vi "ImportConfigFile.vi"(4 "error in (no error)":errorcluster, 5 "bVerify":bool=TRUE, 6 "pszFilePath":string, 7 "nInputHandle":u64) -> (0 "error out":errorcluster, 1 "GX_STATUS":i32, 3 "nOutputHandle":u64)   [LabVIEW 2016, in "GxLVLib.lvlib"]
uses:
  GxLVLib.lvlib
  GxIAPI.dll
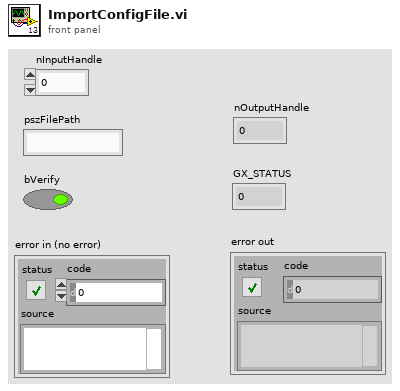
[diagram p1: front panel]
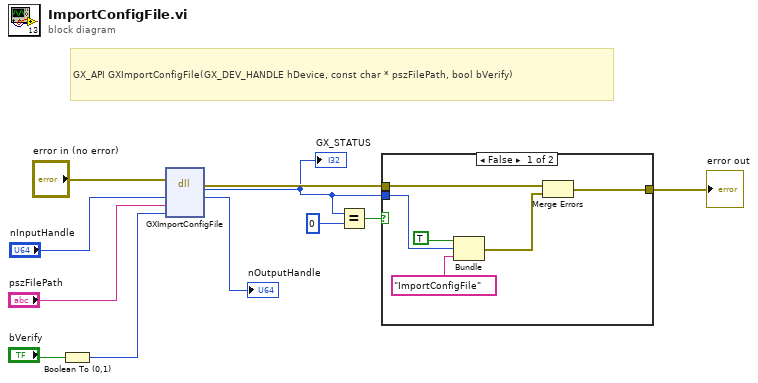
[diagram p0: block diagram]
diagram:
  # "GX_API GXImportConfigFile(GX_DEV_HANDLE hDevice, const char * pszFilePath, bool bVerify)"
  n1 = Boolean To (0,1)(Boolean="bVerify") -> (0, 1=w1:i16)
  n2 = dll-call lib="GxIAPI.dll" fn="GXImportConfigFile"(error in="error in (no error)", "hDevice"="nInputHandle", "pszFilePath"="pszFilePath", "bVerify"=w1) -> (error out=w8:errorcluster, "GX_STATUS"=w6:i32, "hDevice"=→"nOutputHandle":i64)  [unwired: 4 in, 1 out]
  "GX_STATUS" <- w6
  n3 = Equal?(x=w6, y=0) -> (x = y?=w9:bool)
  n4 = case shown="False" w9 {
    tunnel: w8 -> [w17 w18]
    tunnel: [w16 w18] -> w7
    tunnel: w6 -> [w14 _]
    frame False {
      n5 = Bundle(TRUE, "GX_STATUS"=w14, "ImportConfigFile") -> (w15:cluster{bool, "GX_STATUS":i32, string})  [unwired: 1 in]
      n6 = Merge Errors(w17, w15) -> (w16:errorcluster)
    }
    frame True {
    }
  }
  "error out" <- w7
